vi "LLen.vi"(0 "reference in":refnum<class "RedisConnection.lvclass">, 1 "Key":string, 11 "Error In":errorcluster) -> (4 "reference out":refnum<class "RedisConnection.lvclass">, 8 "Length":i64, 15 "Error Out":errorcluster)   [LabVIEW 2020, in "RedisConnection.lvclass"]
doc: "<b>LLEN</b>\n\nReturns the length of the list stored at key. If key does not exist, it is interpreted as an empty list and 0 is returned. An error is returned when the value stored at key is not a list."
uses:
  RedisConnection.lvclass
  RedisConnection.lvclass/RedisConnection.ctl
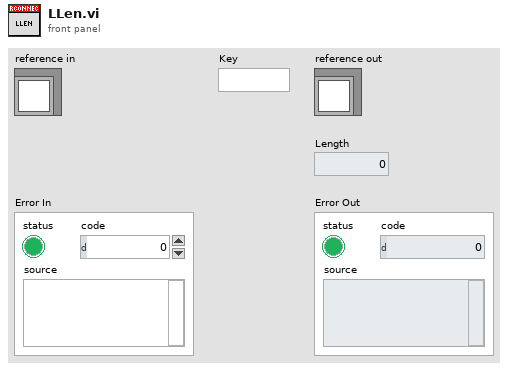
[diagram p1: front panel]
types:
  T1 = typedef "RedisConnection.lvclass/RedisDataType.ctl" = cluster{"Reply Type":T2, "Integer":i64, "String":string, "Multibulk":variant[], "StringData":string[]}
  T2 = typedef "RedisConnection.lvclass/ReplyDataTypeEnum.ctl" = enum16{"None", "Error", "Status", "Nil", "Integer", "String", "Multibulk"}
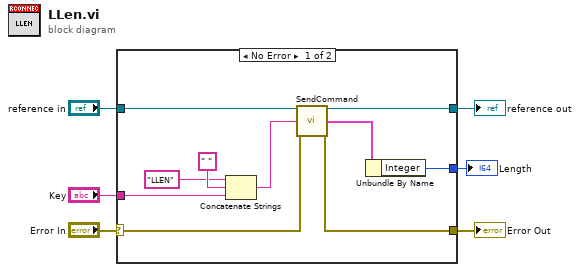
[diagram p0: block diagram]
diagram:
  n1 = case shown="No Error" "Error In" {
    selector: "Error In" -> [w14 w18]
    tunnel: [w13 w18] -> w5
    tunnel: [w16 w17] -> w3
    tunnel: "reference in" -> [w15 w17]
    tunnel: [w7 _] -> w1
    tunnel: "Key" -> [w9 _]
    frame No Error {
      n2 = Concatenate Strings("LLEN", " ", w9) -> (w8:string)
      n3 = call "SendCommand.vi"("reference in"=w15, "Command"=w8, "Error In"=w14) -> ("reference out"=w16:refnum<class "RedisConnection.lvclass">, "Data"=w12:T1, "Error Out"=w13:errorcluster)  [unwired: 10 in]
      n4 = Unbundle By Name(w12) -> ("Integer"=w7:i64)
    }
    frame Error {
    }
  }
  "Error Out" <- w5
  "reference out" <- w3
  "Length" <- w1
